vi "static_response.vi"() -> ()   [LabVIEW 2012]
uses:
  Trace controls.ctl
  probe_point.ctl
  pose_selector.ctl
  pose_source.ctl
  pose_relative_to.ctl
  scan_info.ctl
  <vilib>/Platform/TimedLoop/XDataNode/timing_clust.ctl
  <vilib>/Platform/TimedLoop/XDataNode/nitl_modes.ctl
  <vilib>/Platform/TimedLoop/XDataNode/wakeup.ctl
  <vilib>/Analysis/6fits.llb/Curve Fitting Criteria.ctl
  <vilib>/Platform/TimedLoop/XDataNode/XDataNode.xnode
  <vilib>/Platform/TimedLoop/XDataNode/XDNodeRunTimeDep.lvlib
  <vilib>/Analysis/4window.llb/windowTd.ctl
  <vilib>/Analysis/NI_AALPro.lvlib
  <vilib>/Analysis/4window.llb/Window Properties by Name.vi
  <vilib>/Analysis/4window.llb/Blackman-Harris Window (DBL).vi
panel:
  in  "Plot names":i32(listbox)
  in  "Detrend":bool
  out "Fit display mode":enum32{"Fit off", "Angle", "Moment"}(tab)
  in  "Moment":dbl=1.0
  out "Offset re. moment":dbl format="%#_3p"
  out "Angle (rad)":dbl format="%#_3p"
  out "Angle (deg)":dbl format="%#_3p"
  out "Implied moment (um)":dbl format="%#_3p"
  in  "Sweep unit":enum16{"microns", "mm", "degrees"}(ring) caption="Unit"
  out "Sweep value":dbl caption="Value"
  out "Slope":dbl format="%#_4p"
  out "Calibration (um/V)":dbl=2604.9532508752122
  out "Position":dbl format="%#.2f"
  in  "Calibrate":bool
  out "Raw voltage":dbl format="%#.4f"
  in  "Philtec Sensor":bool
  in  "Line fit":bool
  in  "Pose selectors":T1[](array[typedef])
  out "Response data":dbl[][](array[numeric])
  out "Response plot 2":cluster{"X out":dbl[], dbl[]}[](graph)
  out "XY plot":T4(graph)
  in  "Reference hold":bool
  in  "Responses":cluster{"Individual":bool, "Vector sum":bool}={"Individual"=FALSE, "Vector sum"=TRUE}
  in  "Clear plot":bool
  out "Response plot":cluster{"X out":dbl[], dbl[]}[](graph)
  in  "stop":bool
  in  "Trace controls":T5[](array[typedef])=[{"+ stim"=FALSE, "Relative"=FALSE, "Scale"=enum."1X", "Probe point"=enum."Position (tip)", "XYZ selector"={"Boolean"=FALSE, "Boolean 2"=FALSE, "Boolean 3"=FALSE}, "To tip"=FALSE}, {"+ stim"=FALSE, "Relative"=FALSE, "Scale"=enum."1X", "Probe point"=enum."Position (tip)", "XYZ selector"={"Boolean"=FALSE, "Boolean 2"=FALSE, "Boolean 3"=FALSE}, "To tip"=FALSE}, {"+ stim"=FALSE, "Relative"=FALSE, "Scale"=enum."1X", "Probe point"=enum."Position (tip)", "XYZ selector"={"Boolean"=FALSE, "Boolean 2"=FALSE, "Boolean 3"=FALSE}, "To tip"=FALSE}, {"+ stim"=FALSE, "Relative"=FALSE, "Scale"=enum."1X", "Probe point"=enum."Position (tip)", "XYZ selector"={"Boolean"=FALSE, "Boolean 2"=FALSE, "Boolean 3"=FALSE}, "To tip"=FALSE}]
  # "This VI is used together with sweeper.vi to plot DC responses, mainly from motion sweeps.  Each trace cycle is averaged to a single point.    See narrowband_response.vi for multi-point frequency response.  For chirp or step FFT response, see frequency_response.vi."
  # "The \"static_response_data\" notifier may be used to receive this data at the end of each sweep.   The first column is the sweep \"x\" value and the remaining columns are the response \"y\" values.   If \"Trace continuous\" is on you may get an extra data point at the start of the sweep."
  # "Enable Line Fit to compute angle or moment."
  # "Radians"
  # "Degrees"
  # "Angle:"
  # "Moment"
  # "Offset"
  # "Sweep:"
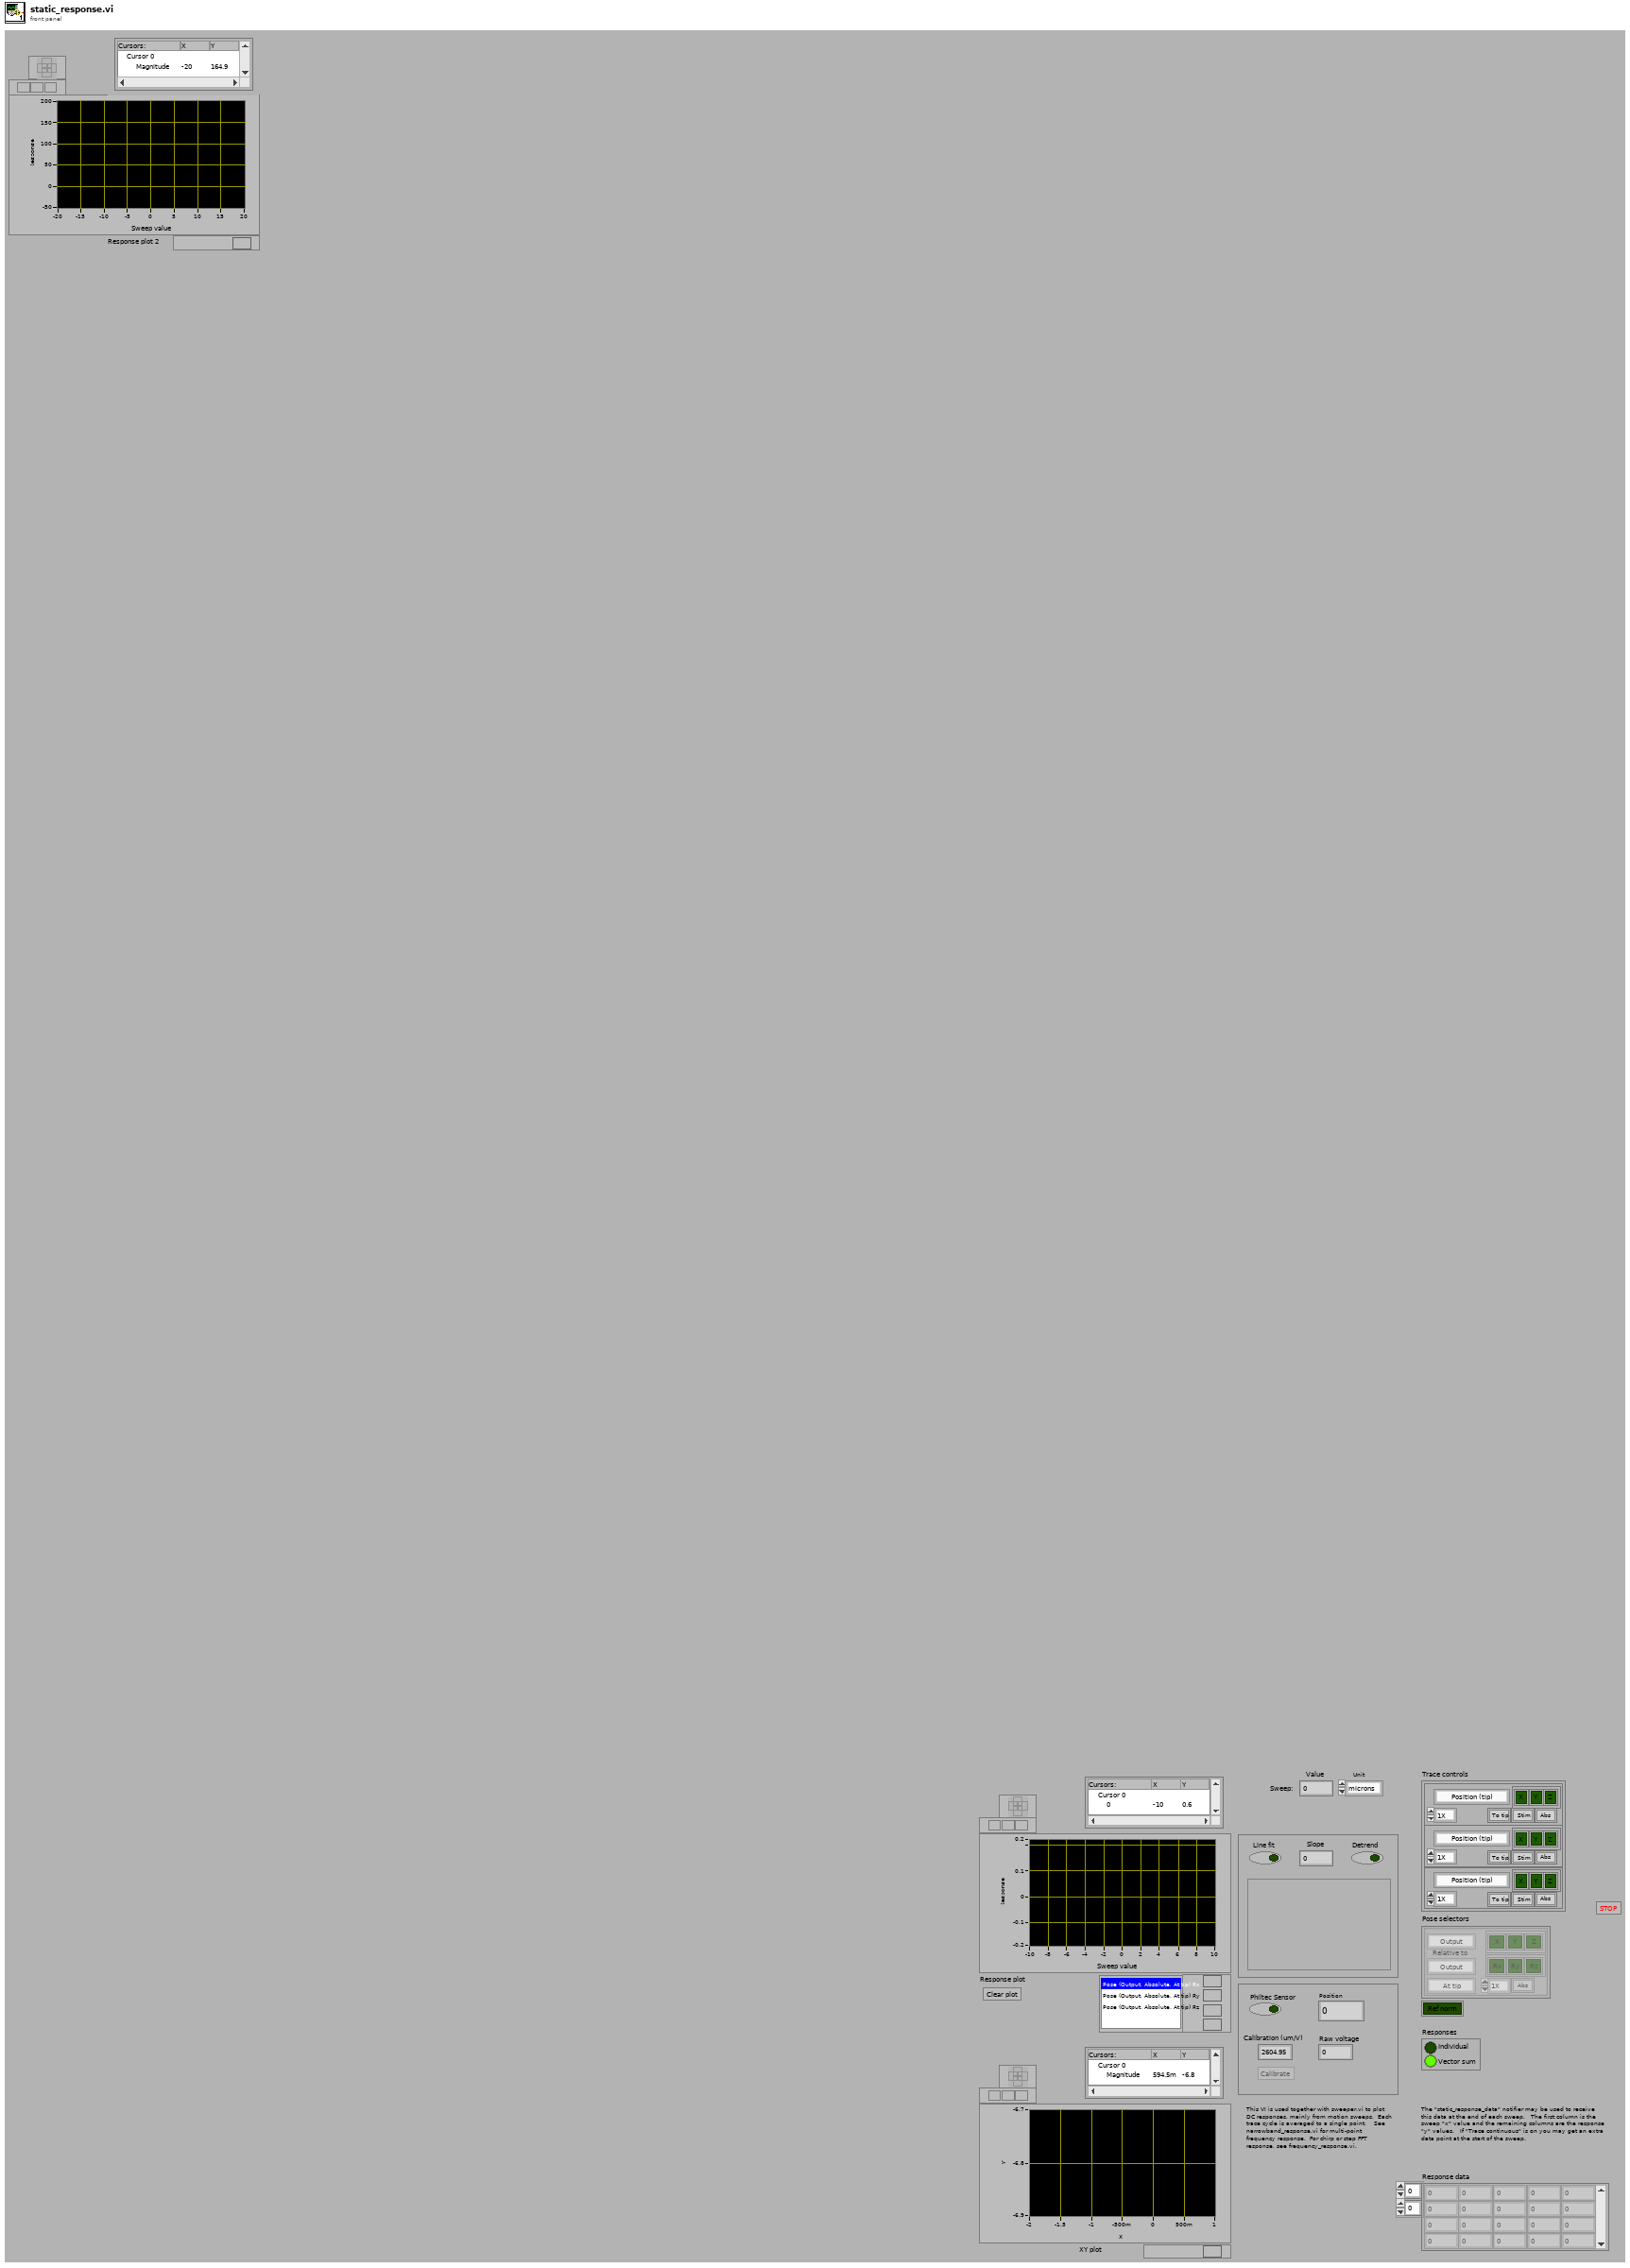
[diagram p1: front panel]
types:
  T1 = typedef "pose_selector.ctl" = cluster{"Scale":enum16{"1X", "10X", "100X", "1KX", "10KX"}, "Source":T2, "XYZ selector":cluster{"Boolean":bool, "Boolean 2":bool, "Boolean 3":bool}, "RPY selector":cluster{"Boolean":bool, "Boolean 2":bool, "Boolean 3":bool}, "Relative to":T3, "Relative":bool, "Translate":enum16{"At tip", "At RCM", "At KC", "At origin"}}
  T2 = typedef "pose_source.ctl" = enum16{"Output", "Handle", "Handle KF", "Goal", "Absolute"}
  T3 = typedef "pose_relative_to.ctl" = enum16{"Output", "Handle", "Handle KF", "Goal", "Absolute", "Trace start"}
  T4 = cluster{"Response data":dbl[], "Response data":dbl[]}
  T5 = typedef "Trace controls.ctl" = cluster{"+ stim":bool, "Relative":bool, "Scale":enum16{"1X", "10X", "100X", "1KX", "10KX"}, "Probe point":T6, "XYZ selector":cluster{"Boolean":bool, "Boolean 2":bool, "Boolean 3":bool}, "To tip":bool}
  T6 = typedef "probe_point.ctl" = enum16{"Position (tip)", "Position (RCM)", "Null pos (tip)", "Null pos (RCM)", "V limiter (tip)", "V Limiter (RCM)", "Goal (tip)", "Goal (RCM)", "Link pos 0", "Link pos 1", "KF link pos 0", "KF link pos 1", "Link rate 0", "Link rate 1", "Link residue 0", "Link residue 1", "Link goal 0", "Link goal 1", "Rate limit 0", "Rate limit 1", "Link error 0", "Link error 1", "Controller 0", "Controller 1", "Output 0", "Output 1", "Drive 0", "Drive 1", "Stimulus 0", "Stimulus 1", "Trace data 0", "Trace data 1", "Analog data 0", "Analog data 1", "Status flags", "Light 0", "Light 1", "Light 2", "Light 3", "Light 4", "Light 5", "Goal origin", "Goal rotation 0", "Goal rotation 1", "Goal rotation 2", "Output origin", "Output rotation 0", "Output rotation 1", "Output rotation 2", "Handle origin", "Handle rotation 0", "Handle rotation 1", "Handle rotation 2", "Handle position", "Handle velocity", "Handle acceleration", "Handle angles", "Handle angle rates", "Handle pos residue", "Handle angle residue", "Trace length"}
  T7 = typedef "scan_info.ctl" = cluster{"Type":enum16{"Frequency", "Offset", "Motion"}, "Start":sgl, "End":sgl, "Npoints":i32}
  T8 = typedef "XDNodeRunTimeDep.lvlib/timing_clust.ctl" = cluster{"Expected End [f-1]":u64, "Actual End [f-1]":u64, "Finished Late? [f-1]":bool, "Expected End [i-1]":u64, "Actual End [i-1]":u64, "Finished Late? [i-1]":bool, "Expected Start [i]":u64, "Actual Start [i]":u64, "Expected Start [f]":u64, "Actual Start [f]":u64, "Source Name":string, "Structure Name":string, "Period":i64, "Deadline":i64, "Offset":i64, "Start":i64, "Priority":i32, "Timeout":i32, "Mode":T9, "Wakeup Reason":T10, "Error":errorcluster, "Source Type":string, "Secondary Source Type":string, "Global End Time":u64, "Global Start Time":u64, "Frame Duration":u64, "Iteration Duration":u64, "Assigned CPU":i32, "I/O Scan Engine Mode":u32}
  T9 = typedef "XDNodeRunTimeDep.lvlib/nitl_modes.ctl" = enum32{"No Change", "Process missed periods, maintain original phase", "Discard missed periods, maintain original phase", "Process missed periods, ignore original phase", "Discard missed periods, ignore original phase"}
  T10 = typedef "XDNodeRunTimeDep.lvlib/wakeup.ctl" = enum32{"Normal", "Aborted", "Asynchronous wakeup", "Timing source error", "Timed loop error", "Timeout"}
  T11 = enum8{"Enabled", "Disabled", "Disabled and Grayed Out"}
  T12 = typedef "NI_AALPro.lvlib/Curve Fitting Criteria.ctl" = u16
  T13 = cluster{"Response data":dbl[], "Best Linear Fit":dbl[]}
  T14 = cluster{"Response data":dbl[], "Best Linear Fit":dbl[]}[]
  T15 = typedef "NI_AALPro.lvlib/windowTd.ctl" = u32
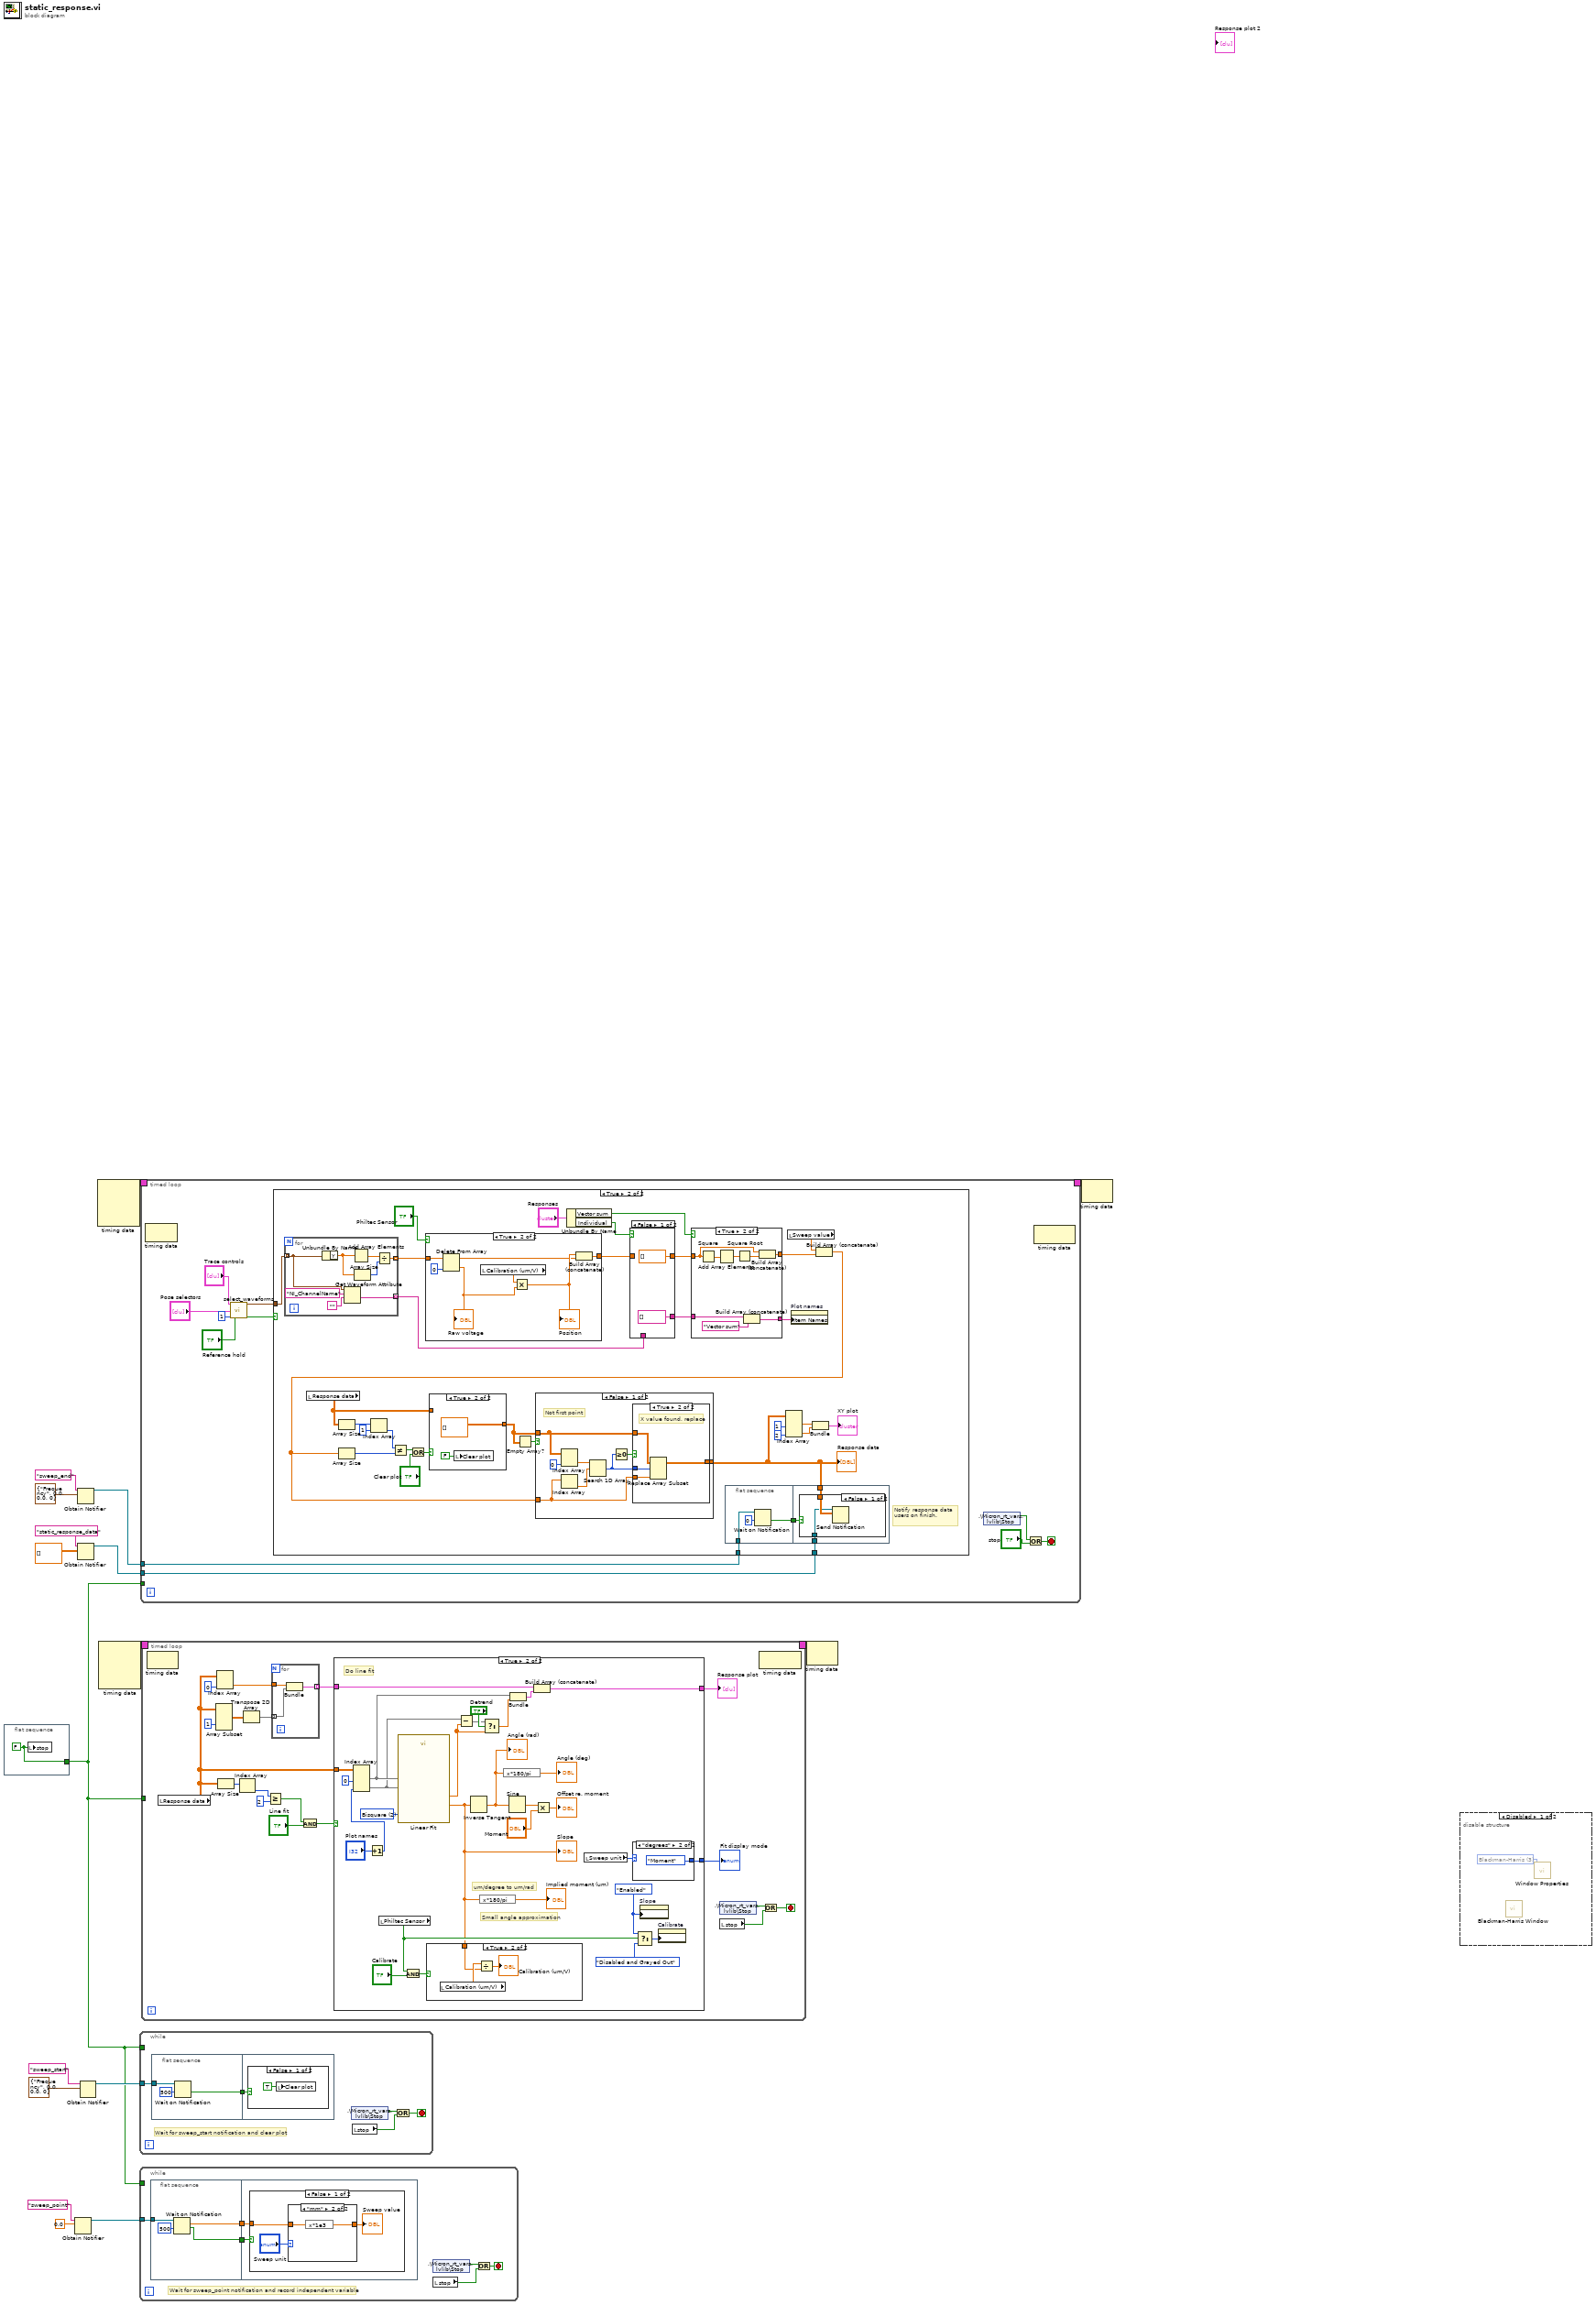
[diagram p0: block diagram]
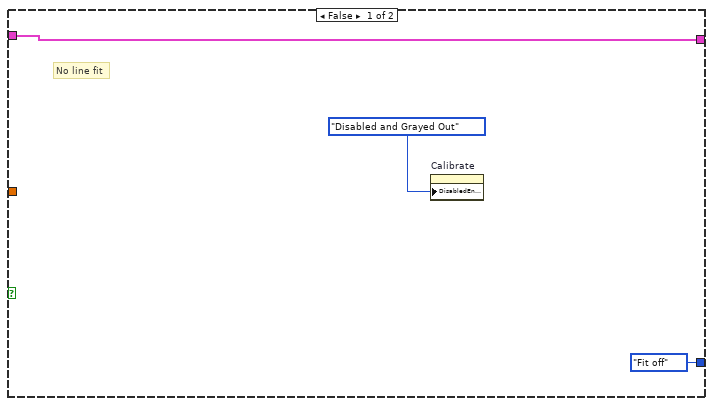
[diagram p2: hidden frame]
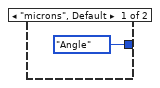
[diagram p3: hidden frame]
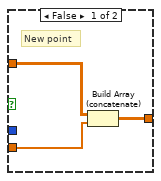
[diagram p13: hidden frame]
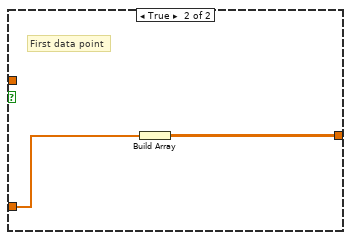
[diagram p14: hidden frame]
diagram:
  n1 = flat-sequence {
    tunnel: [w18] -> w1
    frame #0 {
      w18 = FALSE ("stop")
      n2 = local write "stop"(w18) -> ()
    }
  }
  n3 = Obtain Notifier(name (unnamed)="sweep_point", notification data type=0.0) -> (notifier out=w10:refnum<notifier>)  [unwired: 2 in, 2 out]
  n4 = Obtain Notifier(name (unnamed)="sweep_end", notification data type=T7 {"Type"=enum."Frequency", "Start"=0.0, "End"=0.0, "Npoints"=0} ("Scan Info")) -> (notifier out=w5:refnum<notifier>)  [unwired: 2 in, 2 out]
  n5 = Obtain Notifier(name (unnamed)="static_response_data", notification data type=dbl[][] [] ("transposed array")) -> (notifier out=w4:refnum<notifier>)  [unwired: 2 in, 2 out]
  n6 = Obtain Notifier(name (unnamed)="sweep_start", notification data type=T7 {"Type"=enum."Frequency", "Start"=0.0, "End"=0.0, "Npoints"=0} ("Scan Info")) -> (notifier out=w13:refnum<notifier>)  [unwired: 2 in, 2 out]
  n7 = node-c288() -> (w17:T8)  [unwired: 4 out]
  n8 = node-c288() -> (w3:T8)  [unwired: 4 in]
  n9 = while {
    tunnel: w13 -> [w23]
    tunnel: w1 -> [_]
    stop <- w20 stop-if-true
    # "Wait for sweep_start notification and clear plot"
    n10 = flat-sequence {
      tunnel: w23 -> [w26]
      tunnel: [w24] -> w19
      tunnel: w19 -> [w27]
      frame #0 {
        n11 = Wait on Notification(notifier=w26, timeout in ms (-1)=500) -> (timed out?=w24:bool)  [unwired: 2 in, 3 out]
      }
      frame #1 {
        n12 = case shown="False" w27 {
          frame False {
            n13 = local write "Clear plot"(TRUE ("Clear plot")) -> ()
          }
          frame True {
          }
        }
      }
    }
    n14 = shared-variable ".\\Micron_rt_vars.lvlib\\Stop"() -> (w22:bool)  [unwired: 1 in, 1 out]
    n15 = local read "stop"() -> (w21:bool)
    n16 = Or(x=w22, y=w21) -> (x .or. y?=w20:bool)
  }
  n17 = while {
    tunnel: w10 -> [w34]
    tunnel: w1 -> [_]
    stop <- w31 stop-if-true
    # "Wait for sweep_point notification and record independent variable"
    n18 = flat-sequence {
      tunnel: w34 -> [w38]
      tunnel: [w36] -> w30
      tunnel: [w35] -> w29
      tunnel: w30 -> [w40]
      tunnel: w29 -> [w39]
      frame #0 {
        n19 = Wait on Notification(notifier=w38, timeout in ms (-1)=500) -> (notification=w36:dbl, timed out?=w35:bool)  [unwired: 2 in, 2 out]
      }
      frame #1 {
        n20 = case shown="False" w39 {
          tunnel: w40 -> [w42 _]
          frame False {
            n21 = case shown="\"mm\"" "Sweep unit" {
              tunnel: w42 -> [w44 w46]
              tunnel: [w44 w45] -> w41
              frame "microns", Default {
              }
              frame "mm" {
                n22 = expression code="x*1e3"(w46) -> (w45:dbl)
              }
            }
            "Sweep value" <- w41
          }
          frame True {
          }
        }
      }
    }
    n23 = shared-variable ".\\Micron_rt_vars.lvlib\\Stop"() -> (w33:bool)  [unwired: 1 in, 1 out]
    n24 = local read "stop"() -> (w32:bool)
    n25 = Or(x=w33, y=w32) -> (x .or. y?=w31:bool)
  }
  n26 = timed-loop {
    timing: w17 -> [_]
    timing-out: [_] -> w16
    tunnel: w1 -> [_]
    tunnel: w5 -> [w50]
    tunnel: w4 -> [w49]
    stop <- w54 stop-if-true
    n27 = node-c288() -> ()  [unwired: 2 out]
    n28 = call "select_waveforms.vi"("Trace controls"="Trace controls", "Pose selectors"="Pose selectors", "Decimate"=1, "Reference hold"="Reference hold") -> ("Waveforms out"=w55:waveform(sgl)[], "New data"=w47:bool)  [unwired: 8 in, 2 out]
    n29 = case shown="True" w47 {
      tunnel: w55 -> [_ w85]
      tunnel: w50 -> [_ w83]
      tunnel: w49 -> [_ w66]
      frame False {
      }
      frame True {
        # "Notify response data users on finish."
        n30 = for {
          tunnel: [w146] -> w68 mode=indexing
          tunnel: w85 -> [w144] mode=indexing
          tunnel: [w141] -> w64 mode=indexing
          n31 = Unbundle By Name(w144) -> ("Y"=w145:sgl[])
          n32 = Get Waveform Attribute(5:"", 6:"NI_ChannelName" ("name"), 7:w144) -> (1:w141:string)  [unwired: 1 in, 3 out]
          n33 = Add Array Elements(numeric array=w145) -> (sum=w148:sgl)
          n34 = Array Size(array=w145) -> (size(s)=w147:i32)
          n35 = Divide(x=w148, y=w147) -> (x/y=w146:sgl)
        }
        n36 = local read "Response data"() -> (w79:dbl[][])
        n37 = Array Size(array=w79) -> (size(s)=w82:i32[])
        n38 = Index Array(array=w82, index=1) -> (element=w80:i32)
        n39 = case shown="True" "Philtec Sensor" {
          tunnel: w68 -> [w105 w112]
          tunnel: [w105 w108] -> w63
          frame False {
          }
          frame True {
            n40 = Delete From Array(array=w112, index=0) -> (deleted portion=w109:sgl, array with subset deleted=w106:sgl[])  [unwired: 1 in]
            "Raw voltage" <- w109
            n41 = local read "Calibration (um/V)"() -> (w110:dbl)
            n42 = Multiply(x=w110, y=w109) -> (x*y=w107:dbl)
            "Position" <- w107
            n43 = Build Array (concatenate)(w107, w106) -> (w108:dbl[])
          }
        }
        n44 = Unbundle By Name("Responses") -> ("Vector sum"=w62:bool, "Individual"=w65:bool)
        n45 = case shown="False" w65 {
          tunnel: w64 -> [_ w104]
          tunnel: [string[] [] w104] -> w60
          tunnel: [dbl[] [] w103] -> w61
          tunnel: w63 -> [_ w103]
          frame False {
          }
          frame True {
          }
        }
        n46 = case shown="True" w62 {
          tunnel: w61 -> [w92 w97]
          tunnel: w60 -> [w91 w96]
          tunnel: [w91 w94] -> w58
          tunnel: [w92 w93] -> w59
          frame False {
          }
          frame True {
            n47 = Square(x=w97) -> (x^2=w98:dbl[])
            n48 = Add Array Elements(numeric array=w98) -> (sum=w99:dbl)
            n49 = Square Root(x=w99) -> (sqrt(x)=w100:dbl)
            n50 = Build Array (concatenate)(w96, "Vector sum" ("name")) -> (w94:string[])
            n51 = Build Array (concatenate)(w97, w100) -> (w93:dbl[])
          }
        }
        n52 = flat-sequence {
          tunnel: w83 -> [w132]
          tunnel: [w130] -> w84
          tunnel: w84 -> [w135]
          tunnel: w67 -> [w134]
          tunnel: w66 -> [w133]
          frame #0 {
            n53 = Wait on Notification(notifier=w132, timeout in ms (-1)=0) -> (timed out?=w130:bool)  [unwired: 2 in, 3 out]
          }
          frame #1 {
            n54 = case shown="False" w135 {
              tunnel: w134 -> [w137 _]
              tunnel: w133 -> [w136 _]
              frame False {
                n55 = Send Notification(notification=w137, notifier=w136) -> ()  [unwired: 1 in, 2 out]
              }
              frame True {
              }
            }
          }
        }
        n56 = local read "Sweep value"() -> (w78:dbl)
        n57 = property on="Plot names" class="LstBox (strict)"("Item Names"=w58) -> ()  [unwired: 2 in, 2 out]
        n58 = Build Array (concatenate)(w78, w59) -> (w77:dbl[])
        n59 = Array Size(array=w77) -> (size(s)=w86:i32)
        n60 = Not Equal?(x=w80, y=w86) -> (x != y?=w90:bool)
        n61 = Or(x=w90, y="Clear plot") -> (x .or. y?=w89:bool)
        n62 = case shown="True" w89 {
          tunnel: [w138 dbl[][] [] ("Response data")] -> w75
          tunnel: w79 -> [w138 _]
          frame False {
          }
          frame True {
            n63 = local write "Clear plot"(FALSE ("Clear plot")) -> ()
          }
        }
        n64 = Empty Array?(array=w75) -> (empty?=w76:bool)
        n65 = case shown="False" w76 {
          tunnel: w77 -> [w114 w129]
          tunnel: w75 -> [w115 _]
          tunnel: [w113 w128] -> w67
          frame False {
            # "Not first point"
            n66 = Index Array(array=w115, index (col)=0 ("disabled index (col)")) -> (element=w119:dbl[])  [unwired: 1 in]
            n67 = Index Array(array=w114) -> (element=w118:dbl)  [unwired: 1 in]
            n68 = Search 1D Array(1D array=w119, element=w118) -> (index of element=w116:i32)  [unwired: 1 in]
            n69 = Greater Or Equal To 0?(x=w116) -> (x >= 0?=w117:bool)
            n70 = case shown="True" w117 {
              tunnel: w116 -> [_ w127]
              tunnel: w115 -> [w123 w126]
              tunnel: w114 -> [w122 w125]
              tunnel: [w121 w124] -> w113
              frame False {
                # "New point"
                n71 = Build Array (concatenate)(w123, w122) -> (w121:dbl[][])
              }
              frame True {
                # "X value found, replace"
                n72 = Replace Array Subset(array=w126, new element=w125, index (row)=w127) -> (w124:dbl[][])  [unwired: 1 in]
              }
            }
          }
          frame True {
            # "First data point"
            n73 = Build Array(w129) -> (w128:dbl[][])
          }
        }
        "Response data" <- w67
        n74 = Index Array(array=w67, index (col) #1=1 ("disabled index (col)"), index (col) #2=2 ("index (col)")) -> (element #1=w72:dbl[], element #2=w71:dbl[])  [unwired: 2 in]
        n75 = Bundle("Response data"=w72, "Response data"=w71) -> (→"XY plot":T4)  [unwired: 1 in]
      }
    }
    n76 = shared-variable ".\\Micron_rt_vars.lvlib\\Stop"() -> (w52:bool)  [unwired: 1 in, 1 out]
    n77 = Or(x=w52, y="stop") -> (x .or. y?=w54:bool)
    n78 = node-c288() -> ()  [unwired: 2 out]
  }
  n79 = timed-loop {
    timing: w3 -> [_]
    timing-out: [_] -> w2
    tunnel: w1 -> [_]
    stop <- w153 stop-if-true
    n80 = node-c288() -> ()  [unwired: 1 in, 1 out]
    n81 = local read "Response data"() -> (w158:dbl[][])
    n82 = Array Subset(array=w158, index (col)=1 ("index")) -> (w167:dbl[][])  [unwired: 3 in]
    n83 = Index Array(array=w158, index (col)=0 ("disabled index (col)")) -> (element=w161:dbl[])  [unwired: 1 in]
    n84 = Array Size(array=w158) -> (size(s)=w157:i32[])
    n85 = Index Array(array=w157) -> (element=w156:i32)  [unwired: 1 in]
    n86 = Transpose 2D Array(2D array=w167) -> (transposed array=w168:dbl[][])
    n87 = Greater Or Equal?(x=w156, y=2) -> (x >= y?=w166:bool)
    n88 = for {
      tunnel: w161 -> [w208]
      tunnel: w168 -> [w207] mode=indexing
      tunnel: [w206] -> w162 mode=indexing
      n89 = Bundle("Response data"=w208, w207) -> (w206:cluster{"Response data":dbl[], dbl[]})  [unwired: 1 in]
    }
    n90 = And(x=w166, y="Line fit") -> (x .and. y?=w164:bool)
    n91 = case shown="True" w164 {
      tunnel: w162 -> [w170 w186]
      tunnel: [w170 w198] -> w159
      tunnel: w158 -> [_ w185]
      tunnel: [enum32{"Fit off", "Angle", "Moment"}."Fit off" ("Fit display mode") w179] -> w152
      frame False {
        # "No line fit"
        n92 = property on="Calibrate" class="Bool"("DisabledEnum"=T11."Disabled and Grayed Out" ("Disabled")) -> ()  [unwired: 2 in, 2 out]
      }
      frame True {
        w187 = T12 2 items=["Least Square", "Least Absolute Residual", "Bisquare"] ("method")
        w183 = T11."Enabled" ("Disabled")
        # "Small angle approximation"
        # "um/degree to um/rad"
        # "Do line fit"
        n93 = Increment(x="Plot names") -> (x+1=w172:i32)
        n94 = Index Array(array=w185, index (col) #1=0 ("disabled index (col)"), index (col) #2=w172) -> (element #1=w184:dbl[], element #2=w175:dbl[])  [unwired: 2 in]
        n95 = local read "Philtec Sensor"() -> (w190:bool)
        n96 = call <vilib>:"Linear Fit.vi"("Y"=w175, "X"=w184, "method"=w187) -> ("Best Linear Fit"=w176:dbl[], "slope"=w182:dbl)  [unwired: 8 in, 3 out]
        "Slope" <- w182
        n97 = And(x=w190, y="Calibrate") -> (x .and. y?=w191:bool)
        n98 = case shown="True" w191 {
          tunnel: w182 -> [_ w204]
          frame False {
          }
          frame True {
            n99 = local read "Calibration (um/V)"() -> (w205:dbl)
            n100 = Divide(x=w205, y=w204) -> (x/y=→"Calibration (um/V)":dbl)
          }
        }
        n101 = Subtract(x=w175, y=w176) -> (x-y=w177:dbl[])
        n102 = Inverse Tangent(1:w182) -> (0:w196:dbl)
        "Angle (rad)" <- w196
        n103 = expression code="x*180/pi"(w182) -> (→"Implied moment (um)":dbl)
        n104 = Select(t=w177, s="Detrend", f=w176) -> (s? t:f=w174:dbl[])
        n105 = expression code="x*180/pi"(w196) -> (→"Angle (deg)":dbl)
        n106 = Sine(x=w196) -> (sin(x)=w195:dbl)
        n107 = Bundle("Response data"=w184, "Best Linear Fit"=w174) -> (w199:T13)  [unwired: 1 in]
        n108 = Build Array (concatenate)(w186, w199) -> (w198:T14)
        n109 = Multiply(x=w195, y="Moment") -> (x*y=→"Offset re. moment":dbl)
        n110 = local read "Sweep unit"() -> (w180:enum16{"microns", "mm", "degrees"})
        n111 = case shown="\"degrees\"" w180 {
          tunnel: [enum32{"Fit off", "Angle", "Moment"}."Angle" ("Fit display mode") enum32{"Fit off", "Angle", "Moment"}."Moment" ("Fit display mode")] -> w179
          frame "microns", Default {
          }
          frame "degrees" {
          }
        }
        n112 = Select(t=w183, s=w190, f=T11."Disabled and Grayed Out") -> (s? t:f=w189:T11)
        n113 = property on="Slope" class="DigNum (strict)"("DisabledEnum"=w183) -> ()  [unwired: 2 in, 2 out]
        n114 = property on="Calibrate" class="Bool"("DisabledEnum"=w189) -> ()  [unwired: 2 in, 2 out]
      }
    }
    "Response plot" <- w159
    "Fit display mode" <- w152
    n115 = shared-variable ".\\Micron_rt_vars.lvlib\\Stop"() -> (w154:bool)  [unwired: 1 in, 1 out]
    n116 = local read "stop"() -> (w155:bool)
    n117 = node-c288() -> ()  [unwired: 1 in, 1 out]
    n118 = Or(x=w154, y=w155) -> (x .or. y?=w153:bool)
  }
  n119 = node-c288(w2) -> ()  [unwired: 1 out]
  n120 = node-c288(w16) -> ()  [unwired: 1 out]
  n121 = disable-structure shown="Disabled" {
    frame Disabled {
      w211 = T15 3 items=["Rectangle"=0, "Hanning"=1, "Hamming"=2, "Blackman-Harris"=3, "Exact Blackman"=4, "Blackman"=5, "Flat Top"=6, "4 Term B-Harris "=7, "7 Term B-Harris"=8, "Low Sidelobe"=9, "Blackman Nuttall"=11, "Triangle"=30, "Bartlett-Hanning"=31, "Bohman"=32, "Parzen"=33, "Welch"=34, "Kaiser"=60, "Dolph-Chebyshev"=61, "Gaussian"=62] ("window")
      n122 = call-poly <vilib>:"Blackman-Harris Window.vi"() -> ()  [unwired: 1 in, 2 out]
      n123 = call-poly <vilib>:"Window Properties.vi"("window"=w211) -> ()  [unwired: 8 in, 3 out]
    }
    frame Enabled {
    }
  }
